vi "_RT_CtrlLoop_D999_StrConvValue.vi"(8 "error in (no error)":errorcluster, 10 "Response Str":string) -> (0 "error IO":errorcluster, 2 "appended array":i32[](array[numeric]))   [LabVIEW 2018]
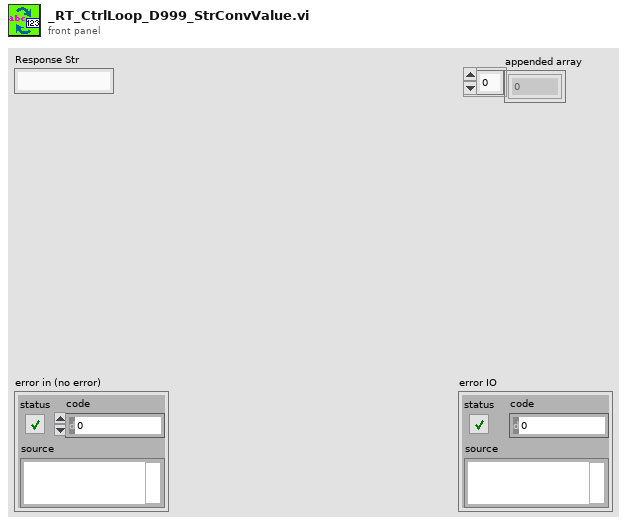
[diagram p1: front panel]
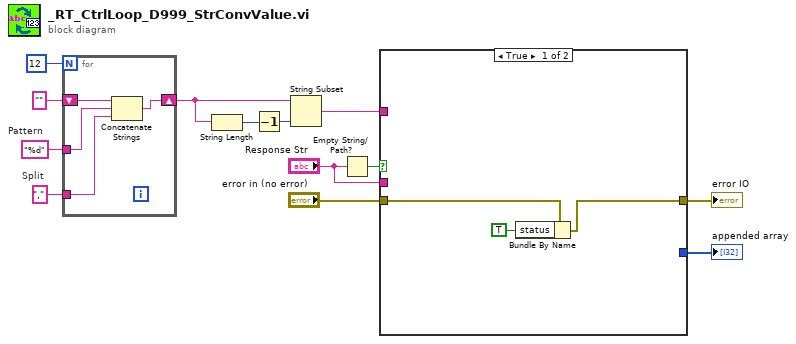
[diagram p0: block diagram]
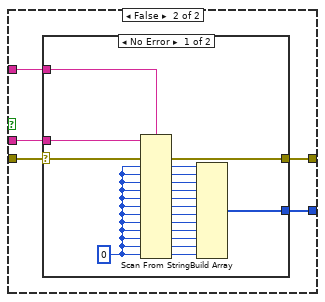
[diagram p2: hidden frame]
diagram:
  w12 = ","  # Split
  w13 = "%d"  # Pattern
  n1 = for {
    N: 12 -> [_]
    tunnel: w13 -> [w16]
    tunnel: w12 -> [w15]
    shift-right: [w14] -> w8
    shift-left: "" -> [w17]
    n2 = Concatenate Strings(w17, w16, w15) -> (w14:string)
  }
  n3 = String Length(string=w8) -> (length=w9:i32)
  n4 = Decrement(x=w9) -> (x-1=w7:i32)
  n5 = String Subset(string=w8, length (rest)=w7) -> (substring=w1:string)  [unwired: 1 in]
  n6 = Empty String/Path?(string/path="Response Str") -> (empty?=w5:bool)
  n7 = case shown="True" w5 {
    tunnel: "Response Str" -> [_ w25]
    tunnel: "error in (no error)" -> [w19 w24]
    tunnel: w1 -> [_ w23]
    tunnel: [w18 w22] -> w6
    tunnel: [_ w21] -> w4
    frame True {
      n8 = Bundle By Name(cluster=w19, "status"=TRUE) -> (w18:errorcluster)
    }
    frame False {
      n9 = case shown="No Error" w24 {
        selector: w24 -> [w29 w44]
        tunnel: w25 -> [w31 _]
        tunnel: w23 -> [w30 _]
        tunnel: [w28 w44] -> w22
        tunnel: [w27 _] -> w21
        frame No Error {
          w26 = 0
          n10 = Scan From String(format string=w30, input string=w31, error in=w29, default 1=w26, default 2=w26, default 3=w26, default 4=w26, default 5=w26, default 6=w26, default 7=w26, default 8=w26, default 9=w26, default 10=w26, default 11=w26, default 12=w26) -> (error out=w28:errorcluster, output 1=w43:i32, output 2=w42:i32, output 3=w41:i32, output 4=w40:i32, output 5=w39:i32, output 6=w38:i32, output 7=w37:i32, output 8=w36:i32, output 9=w35:i32, output 10=w34:i32, output 11=w33:i32, output 12=w32:i32)  [unwired: 1 in, 2 out]
          n11 = Build Array(w43, w42, w41, w40, w39, w38, w37, w36, w35, w34, w33, w32) -> (w27:i32[])
        }
        frame Error {
        }
      }
    }
  }
  "error IO" <- w6
  "appended array" <- w4
